vi "PicoStatus.vi"(1 "PICO STATUS":u32, 2 "error in":errorcluster, 3 "source":string) -> (0 "error out":errorcluster)   [LabVIEW 2020]
doc: "This VI checks the status value returned by calls to the driver. If the driver returns an error, the status member of the error cluster is set to 'true' and the error code and source are set."
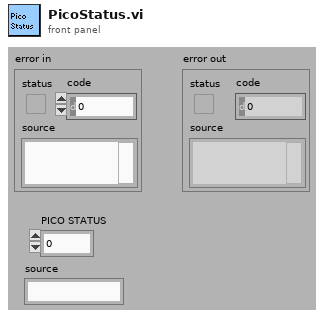
[diagram p1: front panel]
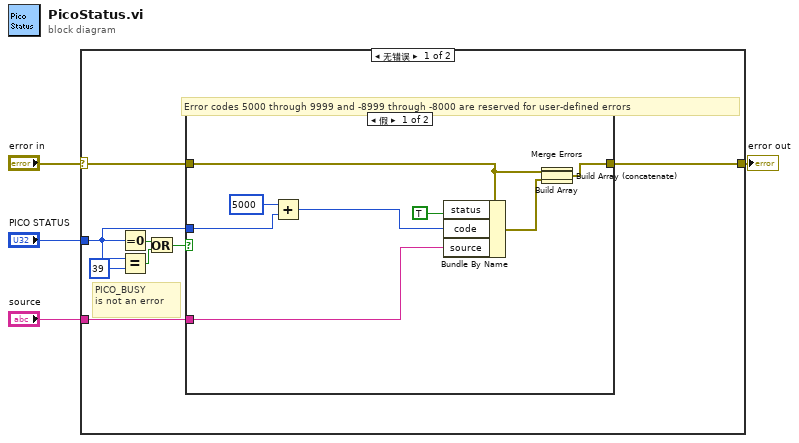
[diagram p0: block diagram]
diagram:
  n1 = case shown="无错误" "error in" {
    selector: "error in" -> [w11 w24]
    tunnel: [w12 w24] -> w4
    tunnel: "PICO STATUS" -> [w6 _]
    tunnel: "source" -> [w10 _]
    frame No Error {
      # "PICO_BUSY \nis not an error"
      # "Error codes 5000 through 9999 and -8999 through -8000 are reserved for user-defined errors"
      n2 = Equal To 0?(x=w6) -> (x = 0?=w9:bool)
      n3 = Equal?(x=w6, y=39) -> (x = y?=w7:bool)
      n4 = Or(x=w9, y=w7) -> (x .or. y?=w8:bool)
      n5 = case shown="假" w8 {
        tunnel: w11 -> [w21 w23]
        tunnel: [w22 w23] -> w12
        tunnel: w6 -> [w20 _]
        tunnel: w10 -> [w15 _]
        frame False {
          n6 = Add(x=5000, y=w20) -> (x+y=w16:u32)
          n7 = Bundle By Name(cluster=w21, "status"=TRUE, "code"=w16, "source"=w15) -> (w19:errorcluster)
          n8 = Build Array(w21, w19) -> (w14:errorcluster[])
          n9 = Build Array (concatenate)(w14) -> (w13:errorcluster[])
          n10 = Merge Errors(w13) -> (w22:errorcluster)
        }
        frame True {
        }
      }
    }
    frame Error {
    }
  }
  "error out" <- w4
